vi "NI VeriStand - Open Fault Manager Reference.vi"(8 "error in (no error)":errorcluster, 11 "Gateway IP Address (\"\": localhost)":string) -> (0 "error out":errorcluster, 3 "ChannelFault":T1)   [LabVIEW 2020, in "NI_VS ChannelFault ExecutionAPI.lvlib"]
doc: "Opens a reference to the channel fault manager on the VeriStand Gateway. You must open a reference before using any other VIs on this palette."
uses:
  <vilib>/NI VeriStand/Execution/ChannelFaultManager/NI_VS ChannelFault ExecutionAPI.lvlib
  <vilib>/NI VeriStand/Execution/ChannelFaultManager/ChannelFaultAPI.ctl
  NationalInstruments.VeriStand.ClientAPI
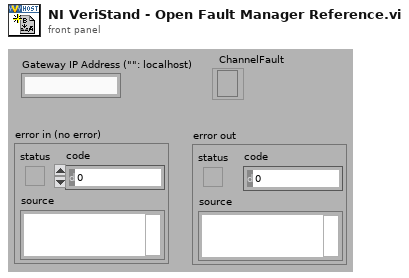
[diagram p1: front panel]
types:
  T1 = typedef "NI_VS ChannelFault ExecutionAPI.lvlib/ChannelFaultAPI.ctl" = refnum<k24>
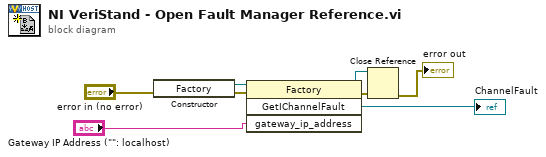
[diagram p0: block diagram]
diagram:
  n1 = constructor class="Factory"(error in="error in (no error)") -> (reference out=w7:refnum<k24>, error out=w8:errorcluster)  [unwired: 2 in, 1 out]
  n2 = invoke class="Factory" method="GetIChannelFault"(reference=w7, error in=w8, "gateway_ip_address"="Gateway IP Address (\"\": localhost)") -> (reference out=w5:refnum<k24>, error out=w6:errorcluster, "GetIChannelFault"=→"ChannelFault":refnum<k24>)  [unwired: 1 in, 1 out]
  n3 = Close Reference(reference=w5, error in (no error)=w6) -> (error out=→"error out":errorcluster)
